vi "Configure Triggered Voltage Level [TRG] Core.vi"(8 "error in (no error)":errorcluster, 9 "triggered level (0.0 Volts)":dbl[unit] format="%^.2e", 10 "channel name (\"CHANNEL1\")":string="CHANNEL1", 11 "CS++DCPwr in":refnum<class "CS++DCPwr.lvclass">) -> (0 "error out":errorcluster, 3 "CS++DCPwr out":refnum<class "CS++DCPwr.lvclass">)   [LabVIEW 2015, in "CS++DCPwr.lvlib" / "CS++DCPwr.lvclass"]
doc: "This VI configures the DC voltage level the power supply attempts to generate after it receives a trigger.\n\nNotes:\n\n(1) This VI is part of the IviDCPwrTrigger [TRG] extension group."
uses:
  CS++DCPwr.lvclass
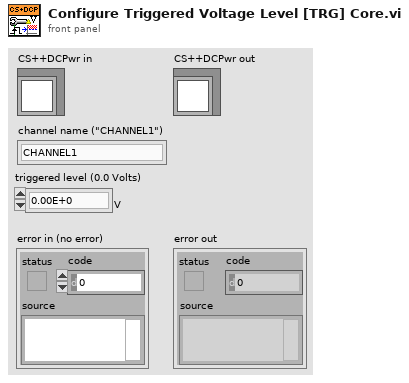
[diagram p1: front panel]
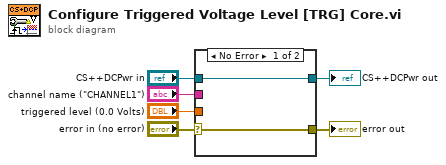
[diagram p0: block diagram]
diagram:
  n1 = case shown="No Error" "error in (no error)" {
    selector: "error in (no error)" -> [w7 w9]
    tunnel: "CS++DCPwr in" -> [w8 w10]
    tunnel: "triggered level (0.0 Volts)" -> [_ _]
    tunnel: "channel name (\"CHANNEL1\")" -> [_ _]
    tunnel: [w7 w9] -> w1
    tunnel: [w8 w10] -> w2
    frame No Error {
    }
    frame Error {
    }
  }
  "error out" <- w1
  "CS++DCPwr out" <- w2
